vi "Sound-Parameters.vi"(4 "Sound Controls":T2={"device ID"=0, "sound format"={"sample rate (S/s)"=44000.0, "number of channels"=2, "bits per sample"=16}, "time (ms)"=200.0}, 7 "Sound Device IN":T4 {"task ID" format="%.0x"}) -> (0 "#samples":u32, 2 "En funcionamiento?":bool, 3 "Sound Device OUT":T4 {"task ID" format="%.0x"})   [LabVIEW 2010]
uses:
  <vilib>/sound2/lvsound2.llb/Sound Output Task ID.ctl
  <vilib>/sound2/lvsound2.llb/Sound Data Format.ctl
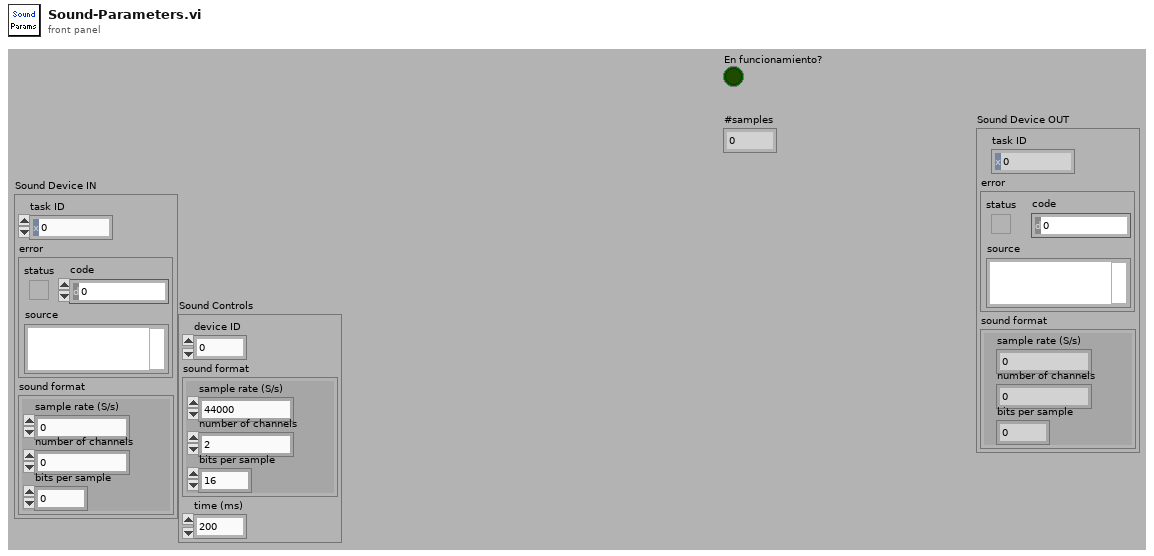
[diagram p1: front panel]
types:
  T1 = typedef "Sound Data Format.ctl" = cluster{"sample rate (S/s)":dbl, "number of channels":i32, "bits per sample":i32}
  T2 = cluster{"device ID":u32, "sound format":T1, "time (ms)":dbl}
  T3 = typedef "Sound Output Task ID.ctl" = u32
  T4 = cluster{"task ID":T3, "error":errorcluster, "sound format":T1}
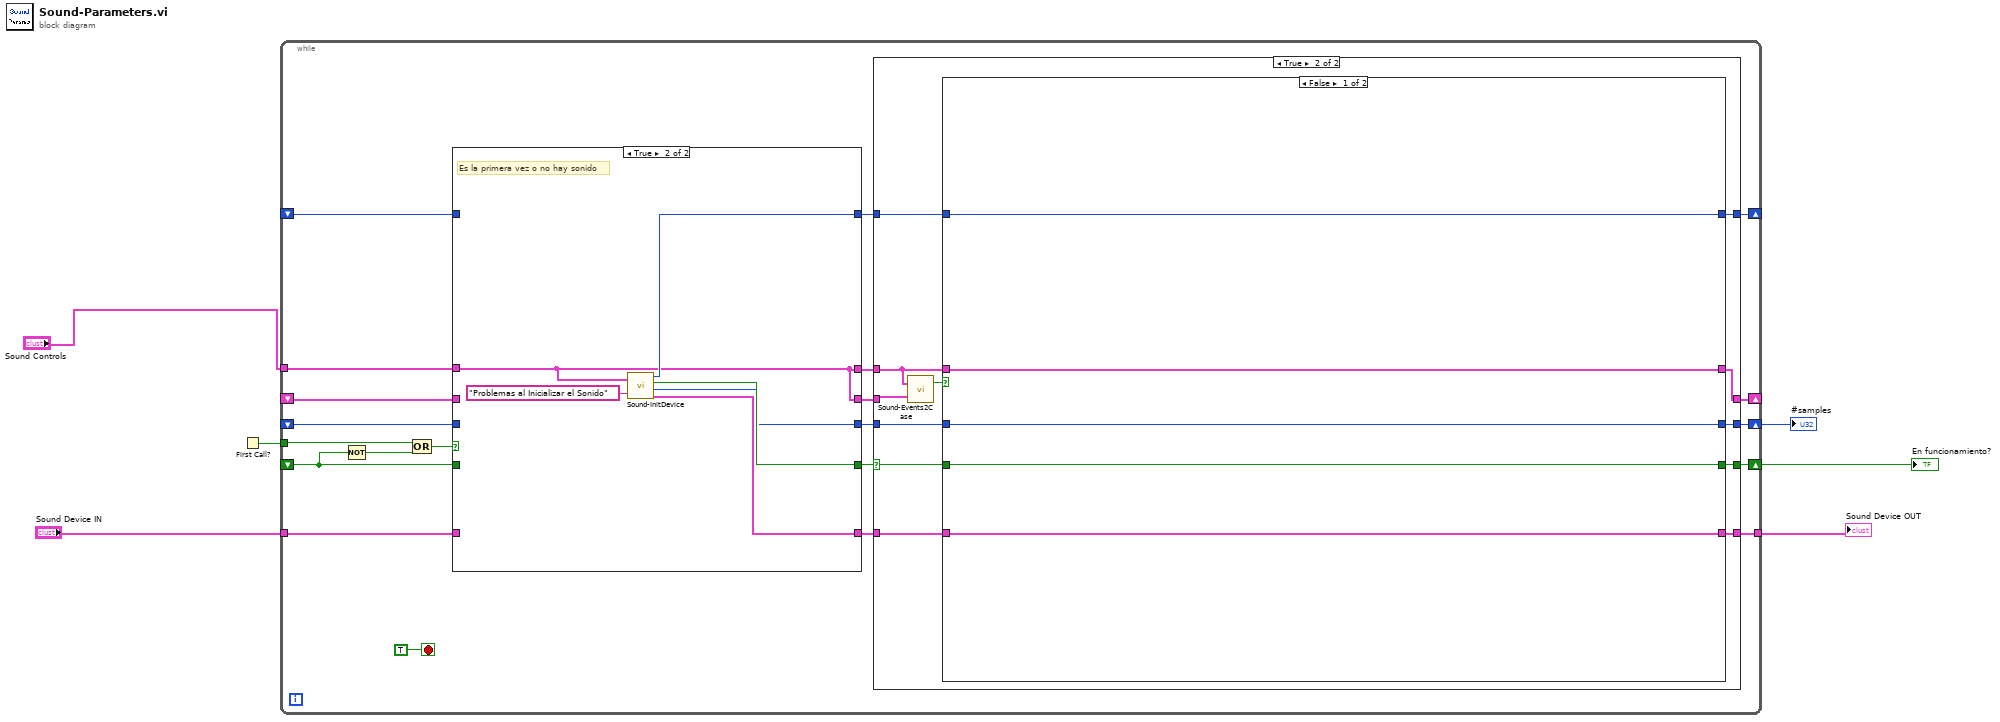
[diagram p0: block diagram]
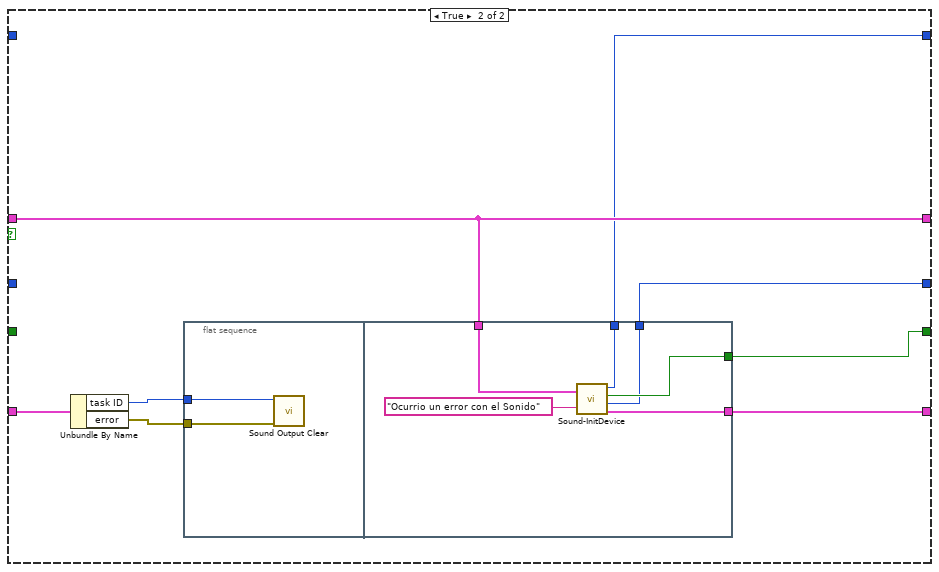
[diagram p3: hidden frame]
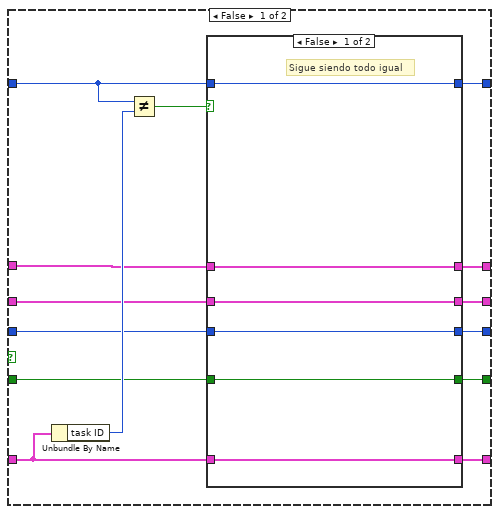
[diagram p4: hidden frame]
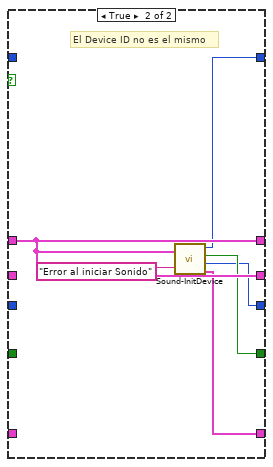
[diagram p5: hidden frame]
diagram:
  n1 = First Call?() -> (First Call?: T/F=w6:bool)
  n2 = while {
    tunnel: "Sound Controls" -> [w23]
    shift-right: [w26] -> _
    shift-left: _ -> [w22]
    tunnel: "Sound Device IN" -> [w14]
    tunnel: [w25] -> w4
    tunnel: w6 -> [w15]
    shift-right: [w16] -> _
    shift-left: _ -> [w19]
    shift-right: [w9] -> w2
    shift-left: _ -> [w7]
    shift-right: [w13] -> w3
    shift-left: _ -> [w11]
    stop <- TRUE stop-if-true
    n3 = Not(x=w7) -> (.not. x?=w8:bool)
    n4 = Compound Arithmetic op=OR(w15, w8) -> (w18:bool)
    n5 = case shown="True" w18 {
      tunnel: [w72 w96] -> w17
      tunnel: [w74 w92] -> w24
      tunnel: w23 -> [w75 w92]
      tunnel: w22 -> [w70 _]
      tunnel: [w73 w92] -> w21
      tunnel: [w79 w97] -> w20
      tunnel: w14 -> [w78 _]
      tunnel: w19 -> [w68 _]
      tunnel: [w71 w95] -> w10
      tunnel: w7 -> [w69 _]
      tunnel: [w67 w94] -> w12
      tunnel: w11 -> [w66 _]
      frame False {
        n6 = Unbundle By Name(w78) -> ("task ID"=w77:T3)
        n7 = Not Equal?(x=w68, y=w77) -> (x != y?=w76:bool)
        n8 = case shown="False" w76 {
          tunnel: [w85 w89] -> w79
          tunnel: w78 -> [w85 _]
          tunnel: w75 -> [w84 w91]
          tunnel: [w84 w91] -> w74
          tunnel: [w83 w91] -> w73
          tunnel: [w81 w90] -> w72
          tunnel: [w82 w88] -> w71
          tunnel: w70 -> [w83 _]
          tunnel: w69 -> [w82 _]
          tunnel: w68 -> [w81 _]
          tunnel: [w80 w87] -> w67
          tunnel: w66 -> [w80 _]
          frame False {
            # "Sigue siendo todo igual"
          }
          frame True {
            # "El Device ID no es el mismo"
            n9 = call "Sound-InitDevice.vi"("Error Message"="Error al iniciar Sonido", "Sound Parameters"=w91) -> ("Sound Device OUT"=w89:T4, "# samples"=w87:u32, "Inizializo?"=w88:bool, "task ID"=w90:T3)
          }
        }
      }
      frame True {
        # "Es la primera vez o no hay sonido"
        n10 = call "Sound-InitDevice.vi"("Error Message"="Problemas al Inicializar el Sonido", "Sound Parameters"=w92) -> ("Sound Device OUT"=w97:T4, "# samples"=w94:u32, "Inizializo?"=w95:bool, "task ID"=w96:T3)
      }
    }
    n11 = case shown="True" w10 {
      selector: w10 -> [w28 w33]
      tunnel: [w32 w43] -> w26
      tunnel: [w31 w42] -> w25
      tunnel: w17 -> [w30 w41]
      tunnel: w24 -> [w32 w38]
      tunnel: w21 -> [_ w37]
      tunnel: w20 -> [w31 w40]
      tunnel: [w30 w39] -> w16
      tunnel: [w29 w36] -> w13
      tunnel: w12 -> [w29 w35]
      tunnel: [w28 w34] -> w9
      frame False {
      }
      frame True {
        n12 = call "Sound-Events2Case.vi"("Sound Controls Old"=w37, "Sound Controls New"=w38) -> ("Sound Cambio?"=w44:bool)  [unwired: 1 out]
        n13 = case shown="False" w44 {
          tunnel: [w49 w53] -> w43
          tunnel: w38 -> [w49 w53]
          tunnel: w40 -> [w48 w57]
          tunnel: [w48 w52] -> w42
          tunnel: w41 -> [w47 _]
          tunnel: [w47 w51] -> w39
          tunnel: [w46 w50] -> w36
          tunnel: w35 -> [w46 _]
          tunnel: [w45 w54] -> w34
          tunnel: w33 -> [w45 _]
          frame False {
          }
          frame True {
            n14 = Unbundle By Name(w57) -> ("task ID"=w55:T3, "error"=w56:errorcluster)
            n15 = flat-sequence {
              tunnel: w55 -> [w59]
              tunnel: w56 -> [w58]
              tunnel: [w63] -> w54
              tunnel: w53 -> [w65]
              tunnel: [w62] -> w52
              tunnel: [w61] -> w51
              tunnel: [w60] -> w50
              frame #0 {
                n16 = call <vilib>:"Sound Output Clear.vi"("error in (no error)"=w58, "task ID"=w59) -> ()  [unwired: 9 in, 1 out]
              }
              frame #1 {
                n17 = call "Sound-InitDevice.vi"("Error Message"="Ocurrio un error con el Sonido" ("message"), "Sound Parameters"=w65) -> ("Sound Device OUT"=w62:T4, "# samples"=w60:u32, "Inizializo?"=w63:bool, "task ID"=w61:T3)
              }
            }
          }
        }
      }
    }
  }
  "Sound Device OUT" <- w4
  "#samples" <- w3
  "En funcionamiento?" <- w2
